vi "Autonomous A3 Right-deliverswitch-move out of way.vi"   [LabVIEW 2017]
uses:
  Framework/Robot Global Data.vi
types:
  T1 = typedef "Command Status Info.ctl" = cluster{"Name":string, "Status":T2, "notifier out":T3}
  T2 = typedef "Completion Status.ctl" = enum16{"Successful", "Aborted", "Incomplete"}
  T3 = typedef "Completion Notifier.ctl" = refnum<notifier>
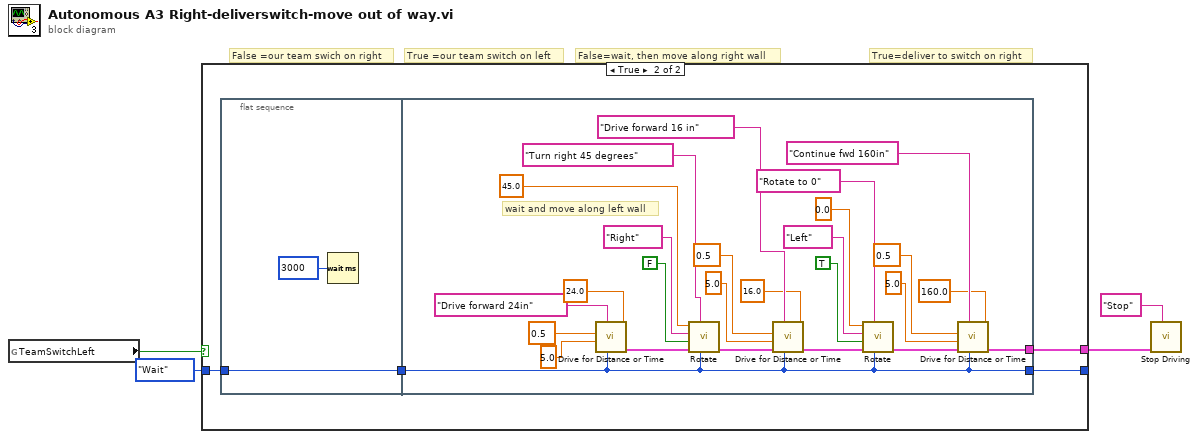
[diagram p0: block diagram]
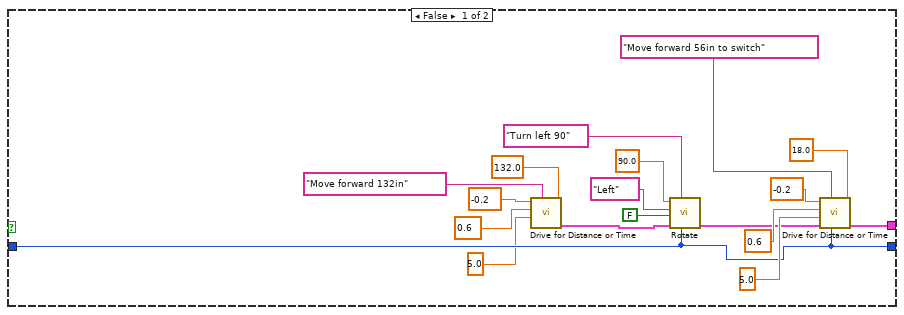
[diagram p2: hidden frame]
diagram:
  # "False=wait, then move along right wall"
  # "True=deliver to switch on right"
  # "False =our team swich on right"
  # "True =our team switch on left"
  n1 = global read "Robot Global Data.vi" "TeamSwitchLeft"() -> (w1:bool)
  n2 = case shown="True" w1 {
    tunnel: [w17 w26] -> w3
    tunnel: [w16 w23] -> _
    tunnel: enum16{"Start", "Wait"}."Wait" ("Synchronication") -> [w16 w25]
    frame False {
      n3 = call "Drive for Distance or Time.vi"("Distance (inches)"=132.0, "Description"="Move forward 132in", "Seconds"=5.0, "Y-axis"=0.6 ("Right Speed"), "X-axis"=-0.2) -> ("Command Info Out"=w7:T1)  [unwired: 6 in]
      n4 = call "Rotate.vi"("Synchronication"=w16, "Description"="Turn left 90", "Command Info In"=w7, "Force Degrees"=FALSE, "Turn Direction"="Left" ("Direction"), "Degrees"=90.0 ("Seconds")) -> ("Command Info Out"=w18:T1)  [unwired: 5 in]
      n5 = call "Drive for Distance or Time.vi"("Distance (inches)"=18.0, "Synchronication"=w16, "Description"="Move forward 56in to switch", "Command Info In"=w18, "Seconds"=5.0, "Y-axis"=0.6 ("Right Speed"), "X-axis"=-0.2) -> ("Command Info Out"=w17:T1)  [unwired: 4 in]
    }
    frame True {
      n6 = flat-sequence {
        tunnel: w25 -> [w28]
        tunnel: [w28] -> w24
        tunnel: [w40] -> w26
        tunnel: w24 -> [w38]
        tunnel: [w38] -> w23
        frame #0 {
          n7 = Wait (ms)(milliseconds to wait=u32 3000) -> ()  [unwired: 1 out]
        }
        frame #1 {
          # "wait and move along left wall"
          n8 = call "Drive for Distance or Time.vi"("Distance (inches)"=24.0, "Synchronication"=w38, "Description"="Drive forward 24in", "Seconds"=5.0, "Y-axis"=0.5 ("Right Speed")) -> ("Command Info Out"=w53:T1)  [unwired: 6 in]
          n9 = call "Rotate.vi"("Synchronication"=w38, "Description"="Turn right 45 degrees", "Command Info In"=w53, "Force Degrees"=FALSE, "Turn Direction"="Right" ("Direction"), "Degrees"=45.0 ("Seconds")) -> ("Command Info Out"=w51:T1)  [unwired: 5 in]
          n10 = call "Drive for Distance or Time.vi"("Distance (inches)"=16.0, "Synchronication"=w38, "Description"="Drive forward 16 in", "Command Info In"=w51, "Seconds"=5.0, "Y-axis"=0.5 ("Right Speed")) -> ("Command Info Out"=w50:T1)  [unwired: 5 in]
          n11 = call "Rotate.vi"("Synchronication"=w38, "Description"="Rotate to 0", "Command Info In"=w50, "Force Degrees"=TRUE, "Turn Direction"="Left" ("Direction"), "Degrees"=0.0 ("Left Speed")) -> ("Command Info Out"=w41:T1)  [unwired: 5 in]
          n12 = call "Drive for Distance or Time.vi"("Distance (inches)"=160.0, "Synchronication"=w38, "Description"="Continue fwd 160in", "Command Info In"=w41, "Seconds"=5.0, "Y-axis"=0.5 ("Right Speed")) -> ("Command Info Out"=w40:T1)  [unwired: 5 in]
        }
      }
    }
  }
  n13 = call "Stop Driving.vi"("Description"="Stop", "Command Info In"=w3) -> ()  [unwired: 9 in, 1 out]
